vi "RedistributePathPoints.vi"(1 "Desired Point Spacing (in)":dbl, 2 "Path Length (in)":dbl, 3 "PathIn":T1[](array[typedef]), 4 "IndexedPathLength":dbl[](array[numeric])) -> (0 "PathOut":T1[](array[typedef]))   [LabVIEW 2017, in "ArgosLib.lvlib"]
uses:
  ArgosLib.lvlib
  TypeDefs/Point2D.ctl
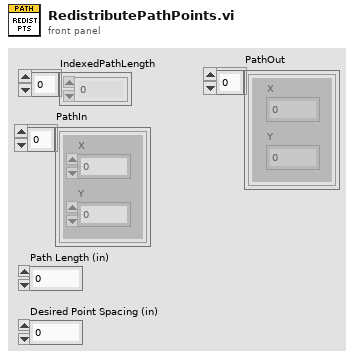
[diagram p1: front panel]
types:
  T1 = typedef "ArgosLib.lvlib/Point2D.ctl" = cluster{"X":dbl, "Y":dbl}
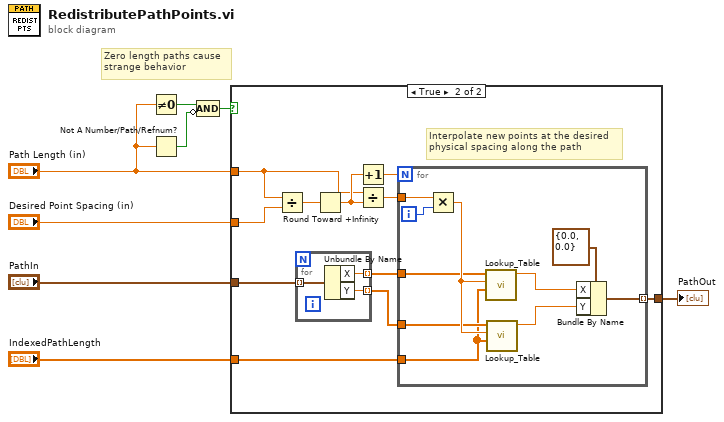
[diagram p0: block diagram]
diagram:
  # "Zero length paths cause\nstrange behavior"
  n1 = Not Equal To 0?(x="Path Length (in)") -> (x != 0?=w4:bool)
  n2 = Not A Number/Path/Refnum?(number/path/refnum="Path Length (in)") -> (NaN/Path/Refnum?=w1:bool)
  n3 = Compound Arithmetic op=AND(w4, invert w1) -> (w3:bool)
  n4 = case shown="True" w3 {
    tunnel: "Desired Point Spacing (in)" -> [_ w20]
    tunnel: "IndexedPathLength" -> [_ w17]
    tunnel: "PathIn" -> [w9 w15]
    tunnel: [w9 w12] -> w5
    tunnel: "Path Length (in)" -> [_ w10]
    frame False {
      # "Zero length path, just pass through"
    }
    frame True {
      # "Interpolate new points at the desired\nphysical spacing along the path"
      n5 = Divide(x=w10, y=w20) -> (x/y=w19:dbl)
      n6 = for {
        tunnel: w15 -> [w23] mode=indexing
        tunnel: [w22] -> w14 mode=indexing
        tunnel: [w21] -> w13 mode=indexing
        n7 = Unbundle By Name(w23) -> ("X"=w22:dbl, "Y"=w21:dbl)
      }
      n8 = Round Toward +Infinity(x=w19) -> (ceil(x): smallest int >= x=w16:dbl)
      n9 = Increment(x=w16) -> (x+1=w11:dbl)
      n10 = Divide(x=w10, y=w16) -> (x/y=w18:dbl)
      n11 = for {
        N: w11 -> [_]
        tunnel: w18 -> [w32]
        tunnel: w14 -> [w30]
        tunnel: w13 -> [w29]
        tunnel: w17 -> [w28]
        tunnel: [w24] -> w12 mode=indexing
        i -> [w33]
        n12 = Multiply(x=w32, y=w33) -> (x*y=w31:dbl)
        n13 = call "Lookup_Table.vi"("Y_Array"=w30, "x_in"=w31, "X_Array"=w28) -> ("y_out"=w26:dbl)  [unwired: 6 in]
        n14 = call "Lookup_Table.vi"("Y_Array"=w29, "x_in"=w31, "X_Array"=w28) -> ("y_out"=w25:dbl)  [unwired: 6 in]
        n15 = Bundle By Name(cluster=T1 {"X"=0.0, "Y"=0.0} ("2DPoint"), "X"=w26, "Y"=w25) -> (w24:T1)
      }
    }
  }
  "PathOut" <- w5
